vi "Aeroflex ATT Set Stimulus.vi"(7 "Aeroflex ATT":T2, 8 "error in (no error)":errorcluster, 10 "ATT Value (dB)":T1, 11 "DAQmx Dev Name (PAModule)":string) -> (0 "error out":errorcluster, 3 "DAQmx Dev Name (PAModule)":string)   [LabVIEW 2011]
uses:
  TypeDefs/Aeroflex ATT Instrument Info.ctl
  tests/Attenuator/TypeDefs/Attenuator ATT Stimulus.ctl
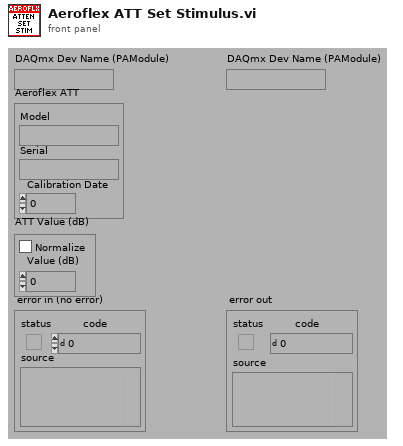
[diagram p1: front panel]
types:
  T1 = typedef "Attenuator ATT Stimulus.ctl" = cluster{"Normalize":bool, "Value (dB)":dbl}
  T2 = typedef "Aeroflex ATT Instrument Info.ctl" = cluster{"Model":string, "Serial":string, "Calibration Date":dbl}
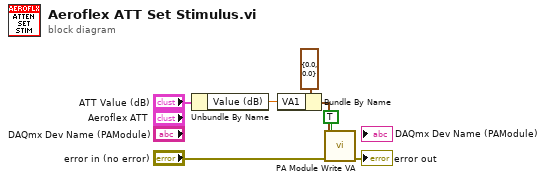
[diagram p0: block diagram]
diagram:
  n1 = Unbundle By Name("ATT Value (dB)") -> ("Value (dB)"=w1:dbl)
  n2 = Bundle By Name(cluster=cluster{"VA1":dbl, "VA2":dbl} {"VA1"=0.0, "VA2"=0.0} ("VA, dB"), "VA1"=w1) -> (w3:cluster{"VA1":dbl, "VA2":dbl})
  n3 = call "PA Module Write VA.vi"("Hardware Present (f)"=TRUE, "error in (no error)"="error in (no error)", "VA, dB"=w3) -> ("error out"=→"error out":errorcluster)  [unwired: 5 in]
